vi "Cond Attr Size.vi"(8 "error in (no error)":errorcluster) -> (0 "error out":errorcluster, 3 "size in memory (bytes)":u64)   [LabVIEW 2013, in "Linux RT IPC.POSIX Threads.lvlib" / "Cond Attr.lvclass"]
doc: "Returns the size in memory for a pthread cond attribute object."
uses:
  Cond Attr.lvclass
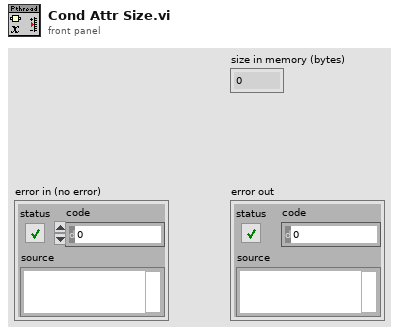
[diagram p1: front panel]
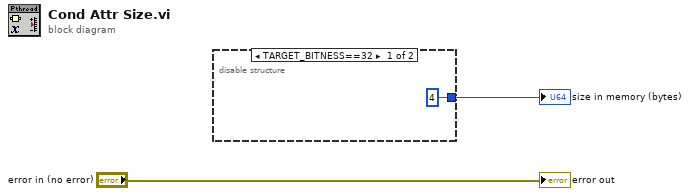
[diagram p0: block diagram]
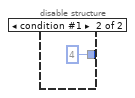
[diagram p2: hidden frame]
diagram:
  n1 = disable-structure shown="TARGET_BITNESS==32" {
    disable-tunnel: [u64 4 ("sem_t size (bytes)") u64 4 ("sem_t size (bytes)")] -> w1
    frame condition #0 (active) {
    }
    frame condition #1 {
    }
  }
  "size in memory (bytes)" <- w1
  "error out" <- "error in (no error)"
